vi "Is Farenheit Mode.vi"(8 "Error In":errorcluster, 11 "Dual Mode Thermometer In":refnum<class "Dual Mode Thermometer.lvclass">) -> (0 "Error Out":errorcluster, 2 "Farenheit Mode":bool, 3 "Dual Mode Thermometer out":refnum<class "Dual Mode Thermometer.lvclass">)   [LabVIEW 2014, in "Dual Mode Thermometer.lvclass"]
doc: "Checks if this thermometer is in Celsius mode (False) or Farenheit mode (True).\n\n\nCopyright (c) 2019 Sze Howe Koh.\nThis code is licensed under the MIT license."
uses:
  Dual Mode Thermometer.lvclass
  Dual Mode Thermometer.lvclass/Dual Mode Thermometer.ctl
  <vilib>/addons/LQ/LQ Core/Qt/CheckState.ctl
  <vilib>/addons/LQ/LQ Core/Qt/Qt.lvlib
  <vilib>/addons/LQ/Qt Widgets/QCheckBox/QCheckBox.lvclass
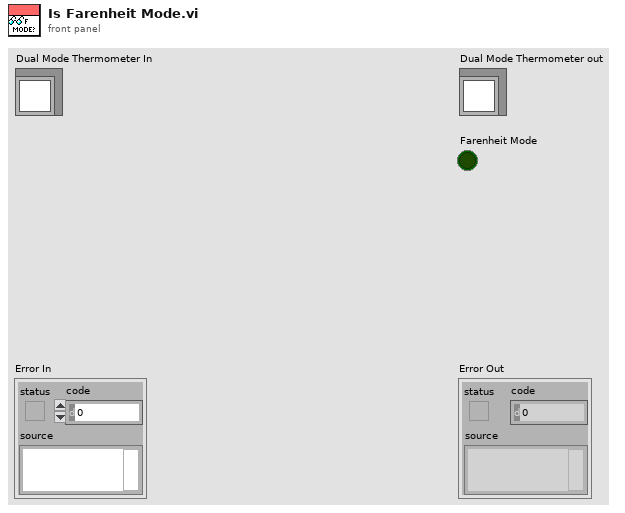
[diagram p1: front panel]
types:
  T1 = typedef "Qt.lvlib/CheckState.ctl" = i32
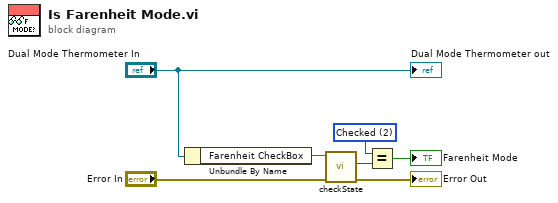
[diagram p0: block diagram]
diagram:
  w1 = T1 2 items=["Unchecked", "PartiallyChecked", "Checked"] ("Value")
  n1 = Unbundle By Name("Dual Mode Thermometer In") -> ("Farenheit CheckBox"=w6:refnum<class "QCheckBox.lvclass">)
  n2 = call <vilib>:"checkState.vi"("Error In"="Error In", "QCheckBox In"=w6) -> ("Error Out"=→"Error Out":errorcluster, "Value"=w5:T1)  [unwired: 7 in, 1 out]
  n3 = Equal?(x=w1, y=w5) -> (x = y?=→"Farenheit Mode":bool)
  "Dual Mode Thermometer out" <- "Dual Mode Thermometer In"
